vi "ExtendedComplex (Scalar) to String.vi"(7 "Use System Default Notation (F)":bool, 11 "Value (CXT)":cxt) -> (3 "Value (String)":string)   [LabVIEW 2013, in "OpenScalar.lvlib"]
uses:
  OpenScalar.lvlib
  FinalStringFormatting.vi
  Get Decimal Separator.vi
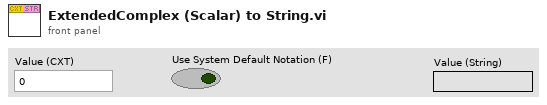
[diagram p1: front panel]
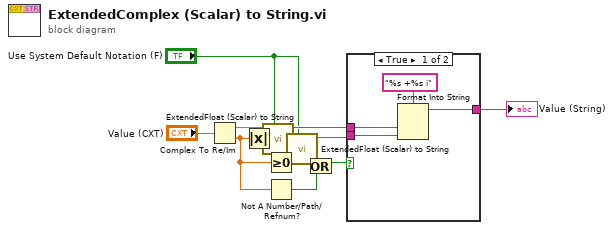
[diagram p0: block diagram]
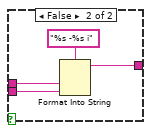
[diagram p2: hidden frame]
diagram:
  n1 = Complex To Re/Im(x + iy="Value (CXT)") -> (x=w3:ext, y=w7:ext)
  n2 = Absolute Value(x=w7) -> (abs(x)=w4:ext)
  n3 = call "ExtendedFloat (Scalar) to String.vi"("Use System Default Notation (F)"="Use System Default Notation (F)", "Value (Extended)"=w3) -> ("Value (String)"=w2:string)  [unwired: 9 in]
  n4 = Greater Or Equal To 0?(x=w7) -> (x >= 0?=w9:bool)
  n5 = Not A Number/Path/Refnum?(number/path/refnum=w7) -> (NaN/Path/Refnum?=w6:bool)
  n6 = call "ExtendedFloat (Scalar) to String.vi"("Use System Default Notation (F)"="Use System Default Notation (F)", "Value (Extended)"=w4) -> ("Value (String)"=w5:string)  [unwired: 9 in]
  n7 = Or(x=w9, y=w6) -> (x .or. y?=w8:bool)
  n8 = case shown="True" w8 {
    tunnel: w2 -> [w15 w19]
    tunnel: w5 -> [w13 w17]
    tunnel: [w12 w16] -> w10
    frame True {
      n9 = Format Into String(format string="%s +%s i", w15, w13) -> (resulting string=w12:string)  [unwired: 2 in, 1 out]
    }
    frame False {
      n10 = Format Into String(format string="%s -%s i", w19, w17) -> (resulting string=w16:string)  [unwired: 2 in, 1 out]
    }
  }
  "Value (String)" <- w10
